vi "Encoder.vi"(8 "Phase B":bool, 9 "Phase A":bool, 11 "CNFG":u8 format="%08b") -> (0 "STAT":u8 format="%08b", 3 "CNTR":u32)   [LabVIEW 2017]
doc: "This VI handles the Encoder Logic with:\n- Input : <b>Phase A</b> and <b>Phase B</b> digital signals and Encoder Configuration (<b>CNFG</b>)\n- Output: Encoder Counter value (<b>CNTR</b>) and Encoder Status (<b>STAT</b>)"
panel:
  # "This VI handles the Encoder Logic with:\n- Input : Phase A and Phase B digital signals and Encoder Configuration (CNFG)\n- Output: Encoder Counter value (CNTR) and Encoder Status (STAT)\n \nThe Encoder Configuration:            The Encoder Status:\nBit 7:5 : Reserved                               Bit 7:6 : Reserved\nBit 4   : Clear Overflow                     Bit 5   : Signed Overflow Error\nBit 3   : Clear Error                             Bit 4   : Unsigned Overflow Error\nBit 2   : Signal Mode                          Bit 3   : Signed Overflow\nBit 1   : Reset                                      Bit 2   : Unsigned Overflow\nBit 0   : Enable                                    Bit 1   : Error in Quad phase mode\n                                                            Bit 0   : Direction"
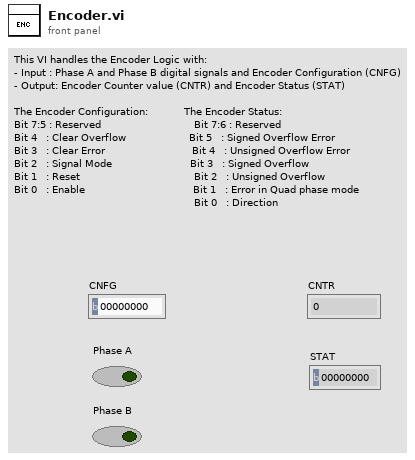
[diagram p1: front panel]
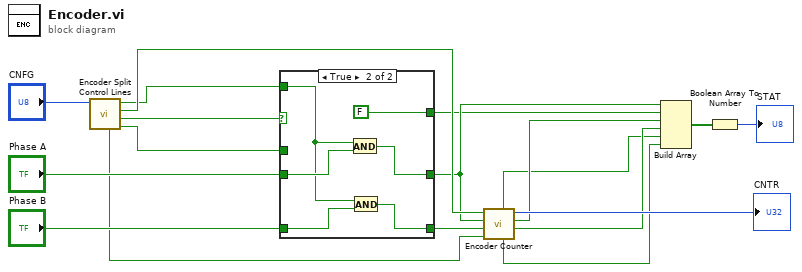
[diagram p0: block diagram]
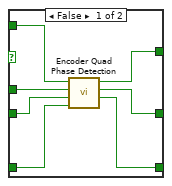
[diagram p2: hidden frame]
diagram:
  n1 = call "Encoder Split Control Lines.vi"("Control"="CNFG") -> ("Clear Error?"=w8:bool, "Dir/Clock Mode?"=w16:bool, "Reset?"=w14:bool, "Enable?"=w9:bool, "Clear Overflow?"=w4:bool)  [unwired: 6 in]
  n2 = case shown="True" w16 {
    tunnel: "Phase A" -> [w24 w31]
    tunnel: "Phase B" -> [w23 w30]
    tunnel: w9 -> [w25 w29]
    tunnel: [w20 FALSE ("Error")] -> w12
    tunnel: [w21 w27] -> w13
    tunnel: [w22 w26] -> w15
    tunnel: w8 -> [w19 _]
    frame False {
      n3 = call "Encoder Quad Phase Detection.vi"("Phase B"=w23, "Phase A"=w24, "Clear Error?"=w19, "Enable?"=w25) -> ("Signal"=w22:bool, "Backward?"=w21:bool, "Error"=w20:bool)  [unwired: 5 in]
    }
    frame True {
      n4 = And(x=w29, y=w31) -> (x .and. y?=w27:bool)
      n5 = And(x=w29, y=w30) -> (x .and. y?=w26:bool)
    }
  }
  n6 = call "Encoder Counter.vi"("Clear Overflow?"=w4, "Signal"=w15, "Backward?"=w13, "Reset?"=w14) -> ("Crossed Halfway?"=w3:bool, "Wrapped around?"=w5:bool, "Count Value"=→"CNTR":u32, "Crossed Halfway twice?"=w1:bool, "Wrapped around twice?"=w2:bool)  [unwired: 3 in]
  n7 = Build Array(w13, w12, w5, w3, w2, w1) -> (w11:bool[])
  n8 = Boolean Array To Number(Boolean array=w11) -> (number=→"STAT":u8)
